vi "Read.vi"(8 "error in (no error)":errorcluster, 11 "Simulated HW in":refnum<class "Simulated HW.lvclass">) -> (0 "error out":errorcluster, 2 "Output":variant, 3 "Simulated HW out":refnum<class "Simulated HW.lvclass">)   [LabVIEW 2017, in "Simulated HW.lvclass"]
uses:
  Simulated HW.lvclass
  C:/Microcellular Plastics Lab/Hardware Settings/Hardware Types/Generic/Generic Hardware.lvclass
  Generic/Generic Hardware.lvclass/Generic Hardware.ctl
  Generic/Accessors/Read Description.vi
  Simulated HW Control Panel.vi
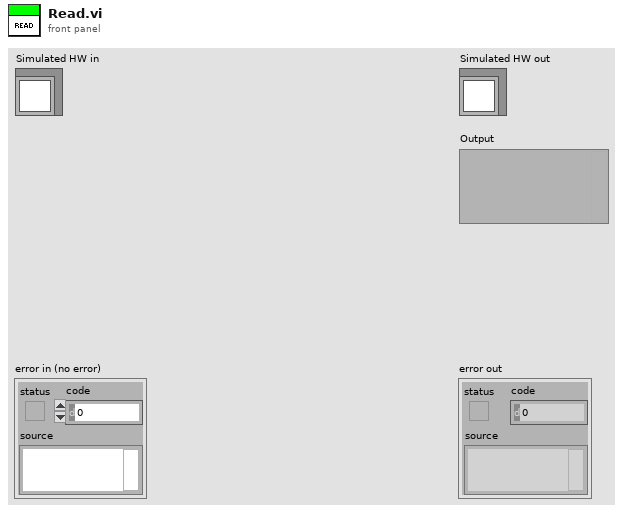
[diagram p1: front panel]
types:
  T1 = typedef "Hardware Settings.lvclass/Hardware Types.ctl" = string
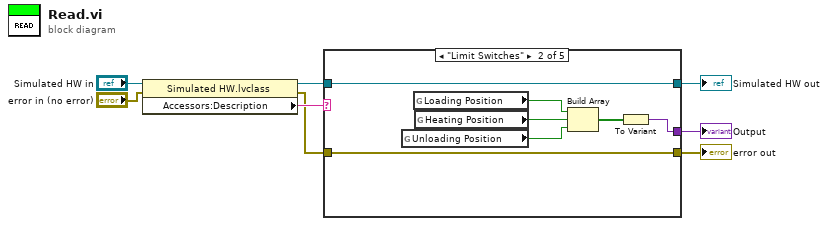
[diagram p0: block diagram]
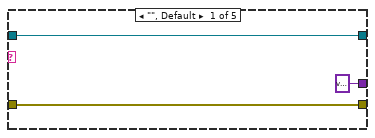
[diagram p2: hidden frame]
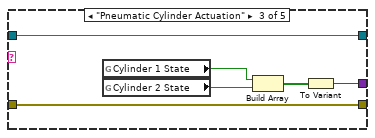
[diagram p3: hidden frame]
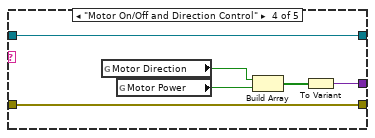
[diagram p4: hidden frame]
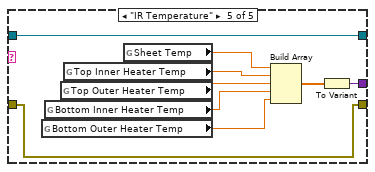
[diagram p5: hidden frame]
diagram:
  n1 = property class="Simulated HW.lvclass"(reference="Simulated HW in", error in="error in (no error)") -> (reference out=w4:refnum<class "Simulated HW.lvclass">, error out=w5:errorcluster, "Accessors:Description"=w6:T1)
  n2 = case shown="\"Limit Switches\"" w6 {
    tunnel: w5 -> [w11 w17 w23 w29 w31]
    tunnel: [w11 w17 w23 w29 w31] -> w1
    tunnel: [w10 w18 w24 w30 w39] -> w3
    tunnel: w4 -> [w10 w18 w24 w30 w39]
    tunnel: [variant ("Variant") w12 w19 w25 w32] -> w2
    frame "", Default {
    }
    frame "Limit Switches" {
      n3 = global read "Simulated HW Control Panel.vi" "Unloading Position"() -> (w14:bool)
      n4 = global read "Simulated HW Control Panel.vi" "Loading Position"() -> (w16:bool)
      n5 = global read "Simulated HW Control Panel.vi" "Heating Position"() -> (w15:bool)
      n6 = Build Array(w16, w15, w14) -> (w13:bool[])
      n7 = To Variant(anything=w13) -> (Variant=w12:variant)
    }
    frame "Pneumatic Cylinder Actuation" {
      n8 = global read "Simulated HW Control Panel.vi" "Cylinder 1 State"() -> (w22:bool)
      n9 = global read "Simulated HW Control Panel.vi" "Cylinder 2 State"() -> (w21:bool)
      n10 = Build Array(w22, w21) -> (w20:bool[])
      n11 = To Variant(anything=w20) -> (Variant=w19:variant)
    }
    frame "Motor On/Off and Direction Control" {
      n12 = global read "Simulated HW Control Panel.vi" "Motor Direction"() -> (w28:bool)
      n13 = global read "Simulated HW Control Panel.vi" "Motor Power"() -> (w27:bool)
      n14 = Build Array(w28, w27) -> (w26:bool[])
      n15 = To Variant(anything=w26) -> (Variant=w25:variant)
    }
    frame "IR Temperature" {
      n16 = global read "Simulated HW Control Panel.vi" "Bottom Outer Heater Temp"() -> (w34:dbl)
      n17 = global read "Simulated HW Control Panel.vi" "Bottom Inner Heater Temp"() -> (w35:dbl)
      n18 = global read "Simulated HW Control Panel.vi" "Top Outer Heater Temp"() -> (w36:dbl)
      n19 = global read "Simulated HW Control Panel.vi" "Top Inner Heater Temp"() -> (w37:dbl)
      n20 = global read "Simulated HW Control Panel.vi" "Sheet Temp"() -> (w38:dbl)
      n21 = Build Array(w38, w37, w36, w35, w34) -> (w33:dbl[])
      n22 = To Variant(anything=w33) -> (Variant=w32:variant)
    }
  }
  "error out" <- w1
  "Simulated HW out" <- w3
  "Output" <- w2
